vi "sort_XY.vi"(10 "sort axis":i32, 11 "Array in":dbl[][](array[numeric])) -> (3 "Array out":dbl[][](array[numeric]))   [LabVIEW 2017]
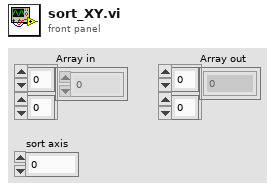
[diagram p1: front panel]
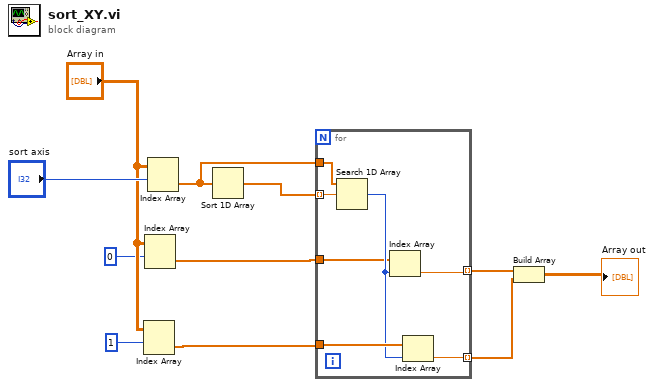
[diagram p0: block diagram]
diagram:
  n1 = Index Array(array="Array in", index (row)=1) -> (element=w7:dbl[])  [unwired: 1 in]
  n2 = Index Array(array="Array in", index (row)=0) -> (element=w9:dbl[])  [unwired: 1 in]
  n3 = Index Array(array="Array in", index (row)="sort axis") -> (element=w2:dbl[])  [unwired: 1 in]
  n4 = Sort 1D Array(array=w2) -> (sorted array=w1:dbl[])
  n5 = for {
    tunnel: [w17] -> w3 mode=indexing
    tunnel: w7 -> [w18]
    tunnel: [w16] -> w4 mode=indexing
    tunnel: w9 -> [w14]
    tunnel: w1 -> [w13] mode=indexing
    tunnel: w2 -> [w12]
    n6 = Search 1D Array(1D array=w12, element=w13) -> (index of element=w15:i32)  [unwired: 1 in]
    n7 = Index Array(array=w14, index=w15) -> (element=w16:dbl)
    n8 = Index Array(array=w18, index=w15) -> (element=w17:dbl)
  }
  n9 = Build Array(w4, w3) -> (→"Array out":dbl[][])
